vi "view ALR_2.vi"(7 "ActivateALRHandling":bool, 9 "ALR_ON_OFF":refnum<data-value>, 10 "ALR_Names":string[][](array[string]), 11 "ALR_State":T1) -> (3 "This VI":refnum<vi>)   [LabVIEW 2019, in "Alarms.lvlib"]
uses:
  Alarms.lvlib
  Ctl/ALRs_State.ctl
panel:
  in  "n_elem":i32(c297)
  out "alrcode":string[](array[string])
  out "alr2":bool
  out "alr1":bool
  out "n alr":i32
  in  "block":bool[](array[boolean])=[FALSE, FALSE, FALSE, FALSE, FALSE, FALSE, FALSE, FALSE, FALSE, FALSE]
  in  "check":bool[](array[boolean])=[FALSE, FALSE, FALSE, FALSE, FALSE, FALSE, FALSE, FALSE, FALSE, FALSE]
  out "alrname":string[](array[string])
  out "t ms view":u32[](array[numeric])
  out "alr view":bool[](array[boolean])
  out "alr not block_view":bool[](array[boolean])
  out "alr on_view":bool[](array[boolean])
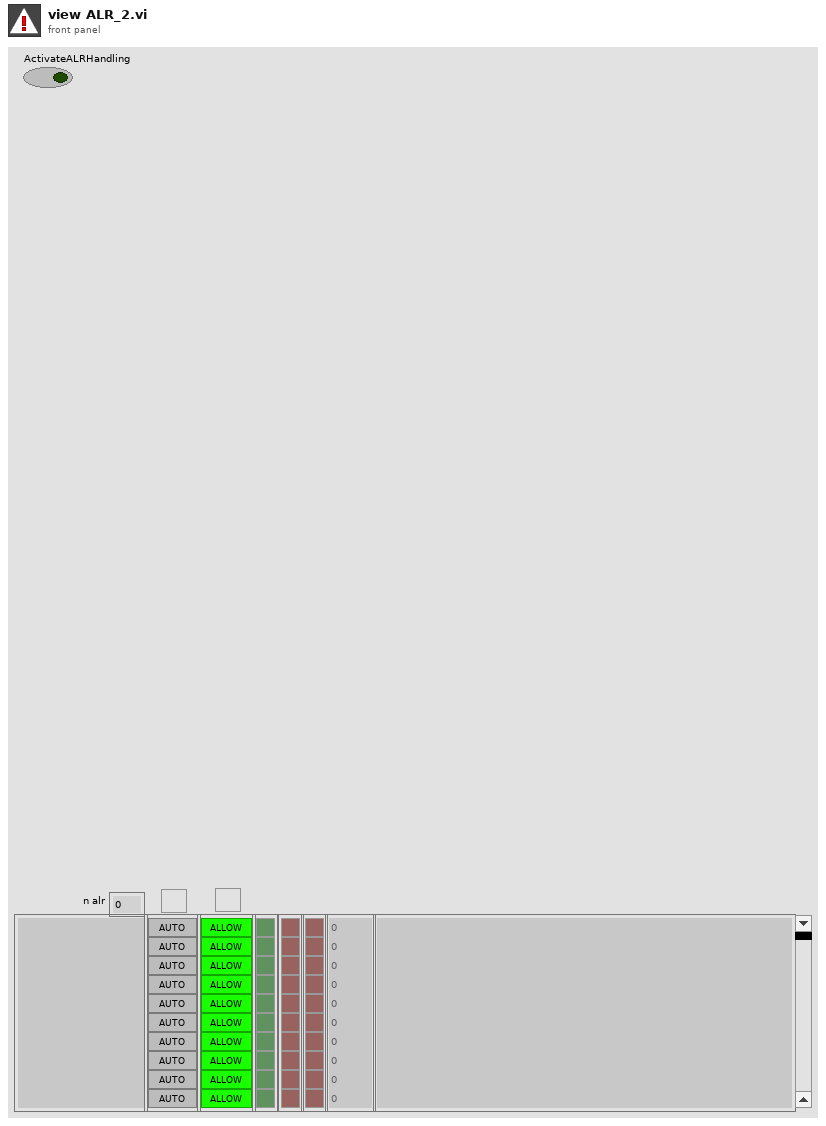
[diagram p1: front panel]
types:
  T1 = typedef "Alarms.lvlib/ALRs_State.ctl" = cluster{"ALR not block":bool[], "ALR":bool[], "ALR blocked":bool[], "ALR ON":bool[], "code":i32[], "level":i32[][], "t ms":u32[], "ack state":enum32{"not", "tripped", "reset", "ack"}[], "color":u32[]}
  T2 = enum32{"Invalid", "Standard", "Closed", "Hidden", "Minimized", "Maximized"}
  T3 = cluster{"ALR_ON":bool[], "ALR_OFF":bool[], "ALR_reset":bool[], "ALR_check":bool[], "ALR_block":bool[], "ALR_Ack":bool[]}
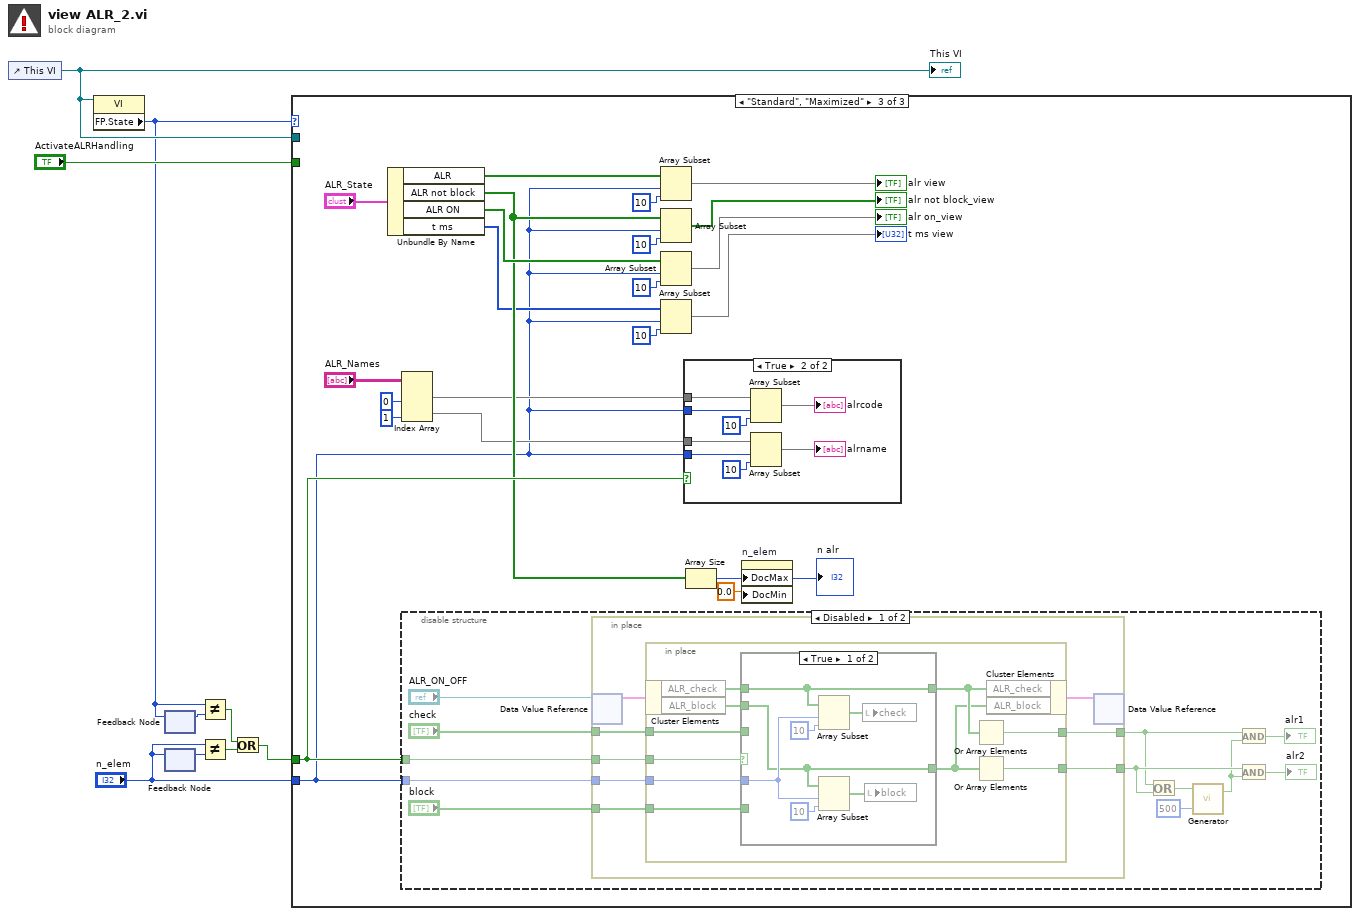
[diagram p0: block diagram]
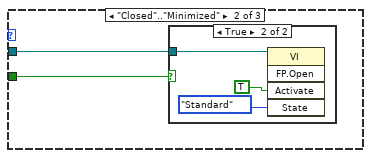
[diagram p3: hidden frame]
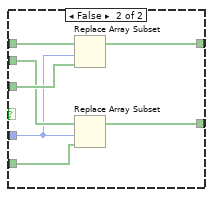
[diagram p5: hidden frame]
diagram:
  n1 = control-ref of="This VI"() -> (w7:refnum<vi>)
  "This VI" <- w7
  n2 = property class="VI"(reference=w7) -> ("FP.State"=w5:T2)  [unwired: 1 in, 2 out]
  n3 = feedback #1() -> (w6:T2)  [unwired: 1 in]
  n4 = feedback-in #1(w5) -> ()
  n5 = feedback #2() -> (w9:i32)  [unwired: 1 in]
  n6 = feedback-in #2("n_elem") -> ()
  n7 = Not Equal?(x=w5, y=w6) -> (x != y?=w4:bool)
  n8 = Not Equal?(x="n_elem", y=w9) -> (x != y?=w3:bool)
  n9 = Or(x=w4, y=w3) -> (x .or. y?=w2:bool)
  n10 = case shown="\"Standard\", \"Maximized\"" w5 {
    tunnel: "ActivateALRHandling" -> [_ w11 _]
    tunnel: w7 -> [_ w10 _]
    tunnel: w2 -> [_ _ w33]
    tunnel: "n_elem" -> [_ _ w15]
    frame "Invalid", Default {
    }
    frame "Closed".."Minimized" {
      n11 = case shown="True" w11 {
        tunnel: w10 -> [_ w12]
        frame False {
        }
        frame True {
          n12 = invoke class="VI" method="FP.Open"(reference=w12, "Activate"=TRUE ("Activate?"), "State"=T2."Standard") -> ()  [unwired: 2 in, 5 out]
        }
      }
    }
    frame "Standard", "Maximized" {
      n13 = Unbundle By Name("ALR_State") -> ("ALR"=w32:bool[], "ALR not block"=w26:bool[], "ALR ON"=w30:bool[], "t ms"=w21:u32[])
      n14 = Index Array(array="ALR_Names", index (col) #1=0 ("disabled index (col)"), index (col) #2=1 ("disabled index (col)")) -> (element #1=w16:string[], element #2=w18:string[])  [unwired: 2 in]
      n15 = disable-structure shown="Disabled" {
        disable-tunnel: w33 -> [w39 _]
        disable-tunnel: w15 -> [w37 _]
        frame Disabled {
          n16 = in-place {
            in-place-border: w37 -> [w54]
            in-place-border: "check" -> [w53]
            in-place-border: "block" -> [w52]
            in-place-border: [w51] -> w45
            in-place-border: [w50] -> w46
            in-place-border: w39 -> [w49]
            n17 = in-place-dvr #3("ALR_ON_OFF") -> (w56:T3)  [unwired: 1 out]
            n18 = in-place {
              in-place-border: w54 -> [w62]
              in-place-border: w53 -> [w65]
              in-place-border: w52 -> [w63]
              in-place-border: [w59] -> w51
              in-place-border: [w58] -> w50
              in-place-border: w49 -> [w57]
              n19 = in-place-cluster #4(w56) -> ("ALR_check"=w66:bool[], "ALR_block"=w64:bool[])
              n20 = case shown="True" w57 {
                tunnel: w66 -> [w72 w79]
                tunnel: w65 -> [_ w80]
                tunnel: w64 -> [w67 w77]
                tunnel: w63 -> [_ w74]
                tunnel: w62 -> [w68 w75]
                tunnel: [w72 w78] -> w61
                tunnel: [w67 w76] -> w60
                frame True {
                  n21 = Array Subset(array=w72, index=w68, length=10) -> (w71:bool[])
                  n22 = Array Subset(array=w67, index=w68, length=10) -> (w69:bool[])
                  n23 = local write "check"(w71) -> ()
                  n24 = local write "block"(w69) -> ()
                }
                frame False {
                  n25 = Replace Array Subset(array=w79, new element=w80, index=w75) -> (w78:bool[])
                  n26 = Replace Array Subset(array=w77, new element=w74, index=w75) -> (w76:bool[])
                }
              }
              n27 = Or Array Elements(Boolean array=w61) -> (logical OR=w59:bool)
              n28 = Or Array Elements(Boolean array=w60) -> (logical OR=w58:bool)
              n29 = in-place-cluster #4("ALR_check"=w61, "ALR_block"=w60) -> (w55:T3)
            }
            n30 = in-place-dvr #3(w55) -> ()  [unwired: 2 out]
          }
          n31 = Or(x=w45, y=w46) -> (x .or. y?=w44:bool)
          n32 = call "Generator.vi"("T ms (500)"=u32 500 ("T (ms)"), "ON (F)"=w44) -> ("Q"=w42:bool)  [unwired: 2 in]
          n33 = And(x=w45, y=w42) -> (x .and. y?=→"alr1":bool)
          n34 = And(x=w46, y=w42) -> (x .and. y?=→"alr2":bool)
        }
        frame Enabled {
        }
      }
      n35 = Array Subset(array=w32, index=w15, length=10) -> (→"alr view":bool[])
      n36 = Array Subset(array=w26, index=w15, length=10) -> (→"alr not block_view":bool[])
      n37 = Array Subset(array=w30, index=w15, length=10) -> (→"alr on_view":bool[])
      n38 = Array Subset(array=w21, index=w15, length=10) -> (→"t ms view":u32[])
      n39 = case shown="True" w33 {
        tunnel: w15 -> [_ w88]
        tunnel: w18 -> [_ w86]
        tunnel: w16 -> [_ w83]
        tunnel: w15 -> [_ w81]
        frame False {
        }
        frame True {
          n40 = Array Subset(array=w83, index=w81, length=10) -> (→"alrcode":string[])
          n41 = Array Subset(array=w86, index=w88, length=10) -> (→"alrname":string[])
        }
      }
      n42 = Array Size(array=w26) -> (size(s)=w35:i32)
      "n alr" <- w35
      n43 = property on="n_elem" class="Scroll (strict)"("DocMax"=w35, "DocMin"=0.0 ("Data Entry Limits:Minimum")) -> ()  [unwired: 2 in, 2 out]
    }
  }
